vi "Station.Initialize.vi"(8 "error in (no error)":errorcluster, 11 "state variables in":T1) -> (0 "error out":errorcluster, 3 "state variables out":T1)   [LabVIEW 2015, in "Overview GUI.lvlib"]
uses:
  Overview GUI.lvlib
  Types/Overview.StateVariables.ctl
  <vilib>/NI Veristand/Execution/Workspace/WorkspaceAPI.ctl
  NationalInstruments.VeriStand.ClientAPI
  <vilib>/NI Veristand/Execution/Workspace/SystemStateRegEventRef.ctl
  <vilib>/NI Veristand/Execution/Workspace/Target State Info.ctl
  <vilib>/NI Veristand/Execution/Workspace/Target State.ctl
  <vilib>/NI Veristand/Execution/Workspace/SystemStateEventRef.ctl
  <vilib>/Utility/miscctls.llb/LVRowAndColumnTypeDef.ctl
  <vilib>/NI/AMC/Queue Registry.vi
  <vilib>/NI/AMC/AMC.lvlib
  <vilib>/NI Veristand/Execution/Workspace/NI_VS Workspace ExecutionAPI.lvlib
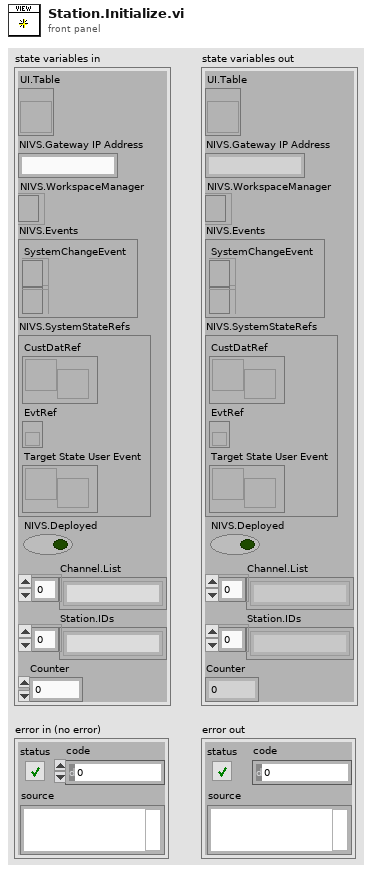
[diagram p1: front panel]
types:
  T1 = typedef "Overview GUI.lvlib/Overview.StateVariables.ctl" = cluster{"UI.Table":refnum<vi>, "NIVS.Gateway IP Address":string, "NIVS.WorkspaceManager":T2, "NIVS.Events":cluster{"SystemChangeEvent":T3, "WorkspaceEvent":refnum<event-registration>}, "NIVS.SystemStateRefs":T4, "NIVS.Deployed":bool, "Channel.List":string[], "Station.IDs":string[], "Counter":u8}
  T2 = typedef "NI_VS Workspace ExecutionAPI.lvlib/WorkspaceAPI.ctl" = refnum<k24>
  T3 = typedef "NI_VS Workspace ExecutionAPI.lvlib/SystemStateRegEventRef.ctl" = refnum<event-registration>
  T4 = typedef "NI_VS Workspace ExecutionAPI.lvlib/SystemStateEventRef.ctl" = cluster{"CustDatRef":refnum<user-event>, "EvtRef":refnum<k27>, "Target State User Event":refnum<user-event>}
  T5 = typedef "LVRowAndColumnTypeDef.ctl" = cluster{"Row":i32, "Column":i32}
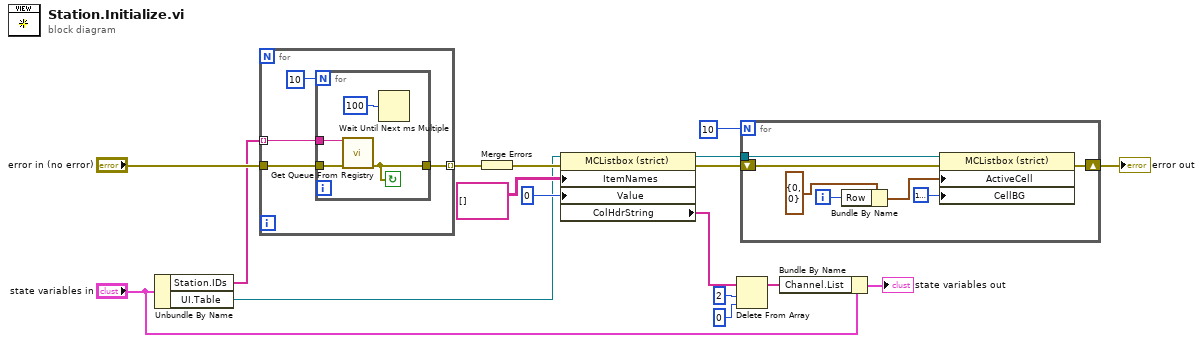
[diagram p0: block diagram]
diagram:
  n1 = Unbundle By Name("state variables in") -> ("Station.IDs"=w13:string[], "UI.Table"=w1:refnum<vi>)
  n2 = for {
    tunnel: w13 -> [w21] mode=indexing
    tunnel: [w19] -> w14 mode=indexing
    tunnel: "error in (no error)" -> [w18]
    n3 = for {
      N: 10 -> [_]
      tunnel: w21 -> [w25]
      tunnel: [w23] -> w19
      tunnel: w18 -> [w22]
      stop <- w23 continue-if-true
      n4 = call <vilib>:"Get Queue From Registry.vi"("name"=w25, "error in"=w22) -> ("error out"=w23:errorcluster)  [unwired: 12 in, 1 out]
      n5 = Wait Until Next ms Multiple(millisecond multiple=u32 100) -> ()  [unwired: 1 out]
    }
  }
  n6 = Merge Errors(w14) -> (w16:errorcluster)
  n7 = property class="MCListbox (strict)"(reference=w1, error in=w16, "ItemNames"=string[][] [] ("Item Names"), "Value"=0) -> (reference out=w10:refnum<vi>, error out=w11:errorcluster, "ColHdrString"=w4:string[])
  n8 = Delete From Array(array=w4, length=2, index=0) -> (array with subset deleted=w7:string[])  [unwired: 1 out]
  n9 = for {
    N: 10 -> [_]
    tunnel: w10 -> [w32]
    shift-right: [w30] -> w17
    shift-left: w11 -> [w31]
    i -> [w26]
    n10 = Bundle By Name(cluster=T5 {"Row"=0, "Column"=0} ("Active Cell:Active Cell"), "Row"=w26) -> (w27:T5)
    n11 = property class="MCListbox (strict)"(reference=w32, error in=w31, "ActiveCell"=w27, "CellBG"=u32 16777216) -> (error out=w30:errorcluster)  [unwired: 1 out]
  }
  "error out" <- w17
  n12 = Bundle By Name(cluster="state variables in", "Channel.List"=w7) -> (→"state variables out":T1)
